vi "ReadData.vi"(8 "error in":errorcluster, 11 "object in":refnum<class "VariantCmd.lvclass">) -> (0 "error out":errorcluster, 2 "Data":variant, 3 "object out":refnum<class "VariantCmd.lvclass">)   [LabVIEW 2020, in "VariantCmd.lvclass"]
doc: "Copyright © 2008 - 2024 VI Technologies B.V. \nALL RIGHTS RESERVED"
uses:
  VariantCmd.lvclass
  VariantCmd.lvclass/VariantCmd.ctl
panel:
  # "Copyright (c) 2024, VI Technologies B.V.\nAll rights reserved.\n\nRedistribution and use in source and binary forms, with or without modification, are permitted provided that \nthe following conditions are met:\n\n * Redistributions of source code must retain the above copyright notice, this list of conditions and the \nfollowing disclaimer.\n * Redistributions in binary form must reproduce the above copyright notice, this list of conditions and the \nfollowing disclaimer in the documentation and/or other materials provided with the distribution.\n * Neither the name of VI Technologies B.V. nor the names of its contributors may be used to endorse or \npromote products derived from this software without specific prior written permission.\n\nTHIS SOFTWARE IS PROVIDED BY THE COPYRIGHT HOLDERS AND CONTRIBUTORS \"AS IS\" AND ANY EXPRESS OR \nIMPLIED WARRANTIES, INCLUDING, BUT NOT LIMITED TO, THE IMPLIED WARRANTIES OF MERCHANTABILITY \nAND FITNESS FOR A PARTICULAR PURPOSE ARE DISCLAIMED. IN NO EVENT SHALL THE COPYRIGHT OWNER OR \nCONTRIBUTORS BE LIABLE FOR ANY DIRECT, INDIRECT, INCIDENTAL, SPECIAL, EXEMPLARY, OR CONSEQUENTIAL \nDAMAGES (INCLUDING, BUT NOT LIMITED TO, PROCUREMENT OF SUBSTITUTE GOODS OR SERVICES; LOSS OF \nUSE, DATA, OR PROFITS; OR BUSINESS INTERRUPTION) HOWEVER CAUSED AND ON ANY THEORY OF LIABILITY, \nWHETHER IN CONTRACT, STRICT LIABILITY, OR TORT (INCLUDING NEGLIGENCE OR OTHERWISE) ARISING IN ANY \nWAY OUT OF THE USE OF THIS SOFTWARE, EVEN IF ADVISED OF THE POSSIBILITY OF SUCH DAMAGE.\n\nFor more information, please visit https://www.vi-tech.nl or contact us at info@vi-tech.nl"
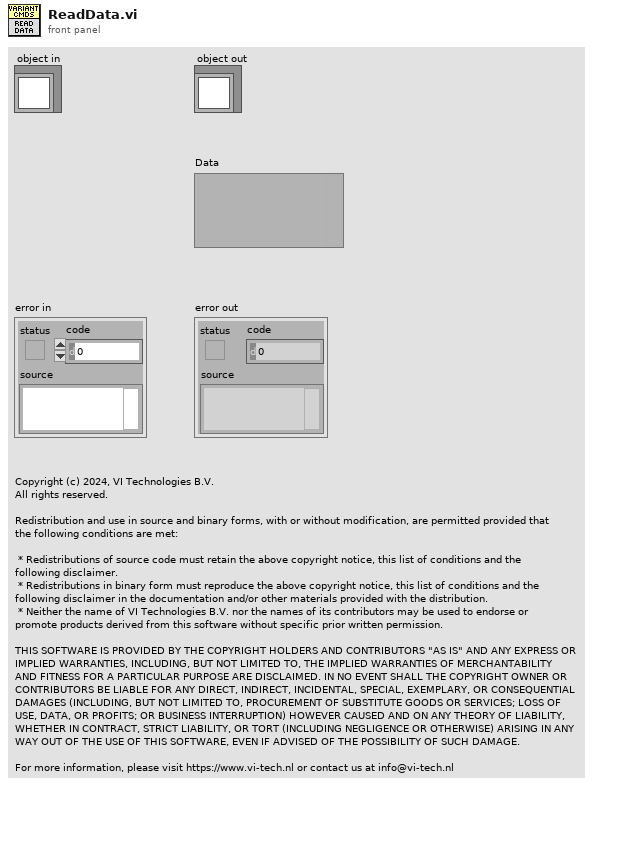
[diagram p1: front panel]
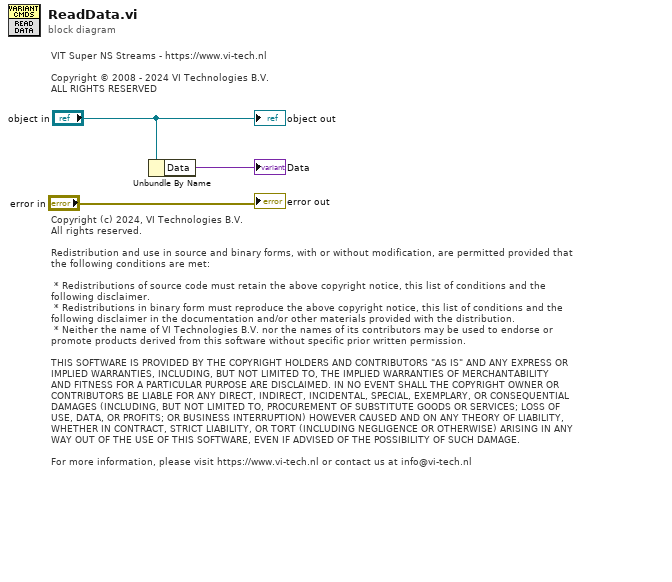
[diagram p0: block diagram]
diagram:
  # "VIT Super NS Streams - https://www.vi-tech.nl\n\nCopyright © 2008 - 2024 VI Technologies B.V. \nALL RIGHTS RESERVED"
  # "Copyright (c) 2024, VI Technologies B.V.\nAll rights reserved.\n\nRedistribution and use in source and binary forms, with or without modification, are permitted provided that \nthe following conditions are met:\n\n * Redistributions of source code must retain the above copyright notice, this list of conditions and the \nfollowing disclaimer.\n * Redistributions in binary form must reproduce the above copyright notice, this list of conditions and the \nfollowing disclaimer in the documentation and/or other materials provided with the distribution.\n * Neither the name of VI Technologies B.V. nor the names of its contributors may be used to endorse or \npromote products derived from this software without specific prior written permission.\n\nTHIS SOFTWARE IS PROVIDED BY THE COPYRIGHT HOLDERS AND CONTRIBUTORS \"AS IS\" AND ANY EXPRESS OR \nIMPLIED WARRANTIES, INCLUDING, BUT NOT LIMITED TO, THE IMPLIED WARRANTIES OF MERCHANTABILITY \nAND FITNESS FOR A PARTICULAR PURPOSE ARE DISCLAIMED. IN NO EVENT SHALL THE COPYRIGHT OWNER OR \nCONTRIBUTORS BE LIABLE FOR ANY DIRECT, INDIRECT, INCIDENTAL, SPECIAL, EXEMPLARY, OR CONSEQUENTIAL \nDAMAGES (INCLUDING, BUT NOT LIMITED TO, PROCUREMENT OF SUBSTITUTE GOODS OR SERVICES; LOSS OF \nUSE, DATA, OR PROFITS; OR BUSINESS INTERRUPTION) HOWEVER CAUSED AND ON ANY THEORY OF LIABILITY, \nWHETHER IN CONTRACT, STRICT LIABILITY, OR TORT (INCLUDING NEGLIGENCE OR OTHERWISE) ARISING IN ANY \nWAY OUT OF THE USE OF THIS SOFTWARE, EVEN IF ADVISED OF THE POSSIBILITY OF SUCH DAMAGE.\n\nFor more information, please visit https://www.vi-tech.nl or contact us at info@vi-tech.nl"
  n1 = Unbundle By Name("object in") -> ("Data"=→"Data":variant)
  "error out" <- "error in"
  "object out" <- "object in"
